vi "Swerve Wheel.vi"(8 "Wheel Angle Offset":dbl, 9 "Inputs":dbl[](array[numeric]), 10 "Pot Ref In":T1, 11 "Wheel":T3(ring)) -> (0 "Pot Ref Out":T1, 1 "Motor Output":dbl, 2 "Wheel Angle":dbl, 3 "Speed":dbl)   [LabVIEW 2018]
uses:
  <vilib>/Rock Robotics/WPI/Potentiometer/WPI_PotentiometerDevRef.ctl
  <vilib>/Rock Robotics/SystemInterfaces/AI/FPGA_AIChannel.ctl
  Drive Train Global.vi
  <vilib>/addons/control/pid/pid.llb/PID (DBL).vi
  <vilib>/addons/control/pid/NI_PID_pid.lvlib
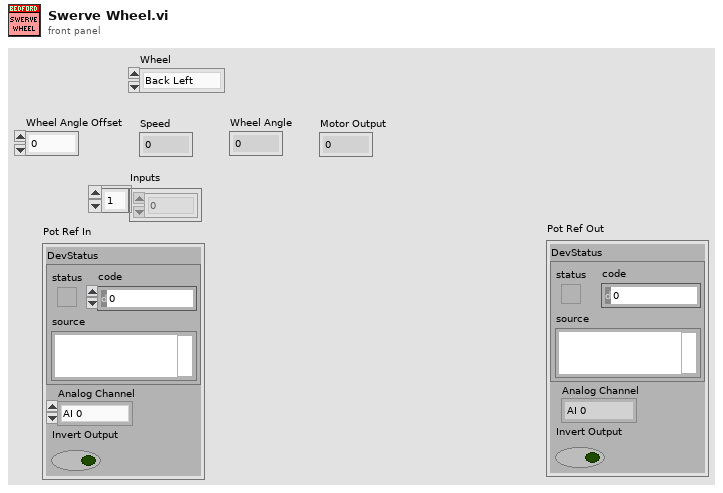
[diagram p1: front panel]
types:
  T1 = typedef "WPI_PotentiometerDevRef.ctl" = cluster{"DevStatus":errorcluster, "Analog Channel":T2, "Invert Output":bool}
  T2 = typedef "FPGA_AIChannel.ctl" = enum8{"AI 0", "AI 1", "AI 2", "AI 3", "AI MXP 0", "AI MXP 1", "AI MXP 2", "AI MXP 3", "Invalid"}
  T3 = enum16{"Back Left", "Back Right", "Front Left", "Front Right"}
  T4 = cluster{"proportional gain (Kc)":dbl, "integral time (Ti, min)":dbl, "derivative time (Td, min)":dbl}
  T5 = enum16{"Z", "Y", "X", "Rot. Point X", "Rot. Point Y", "Width/2", "Max", "Length/2"}
  T6 = enum16{"Z Axis", "Y", "X", "Rot. Point X", "Rot. Point Y", "Width/2", "Max", "Length/2"}
  T7 = cluster{"Front Left":cluster{"P Value":dbl, "I Value":dbl, "D Value":dbl}, "Front Right":cluster{"P Value":dbl, "I Value":dbl, "D Value":dbl}, "Back Left":cluster{"P Value":dbl, "I Value":dbl, "D Value":dbl}, "Back Right":cluster{"P Value":dbl, "I Value":dbl, "D Value":dbl}}
  T8 = cluster{"P Value":dbl, "I Value":dbl, "D Value":dbl}
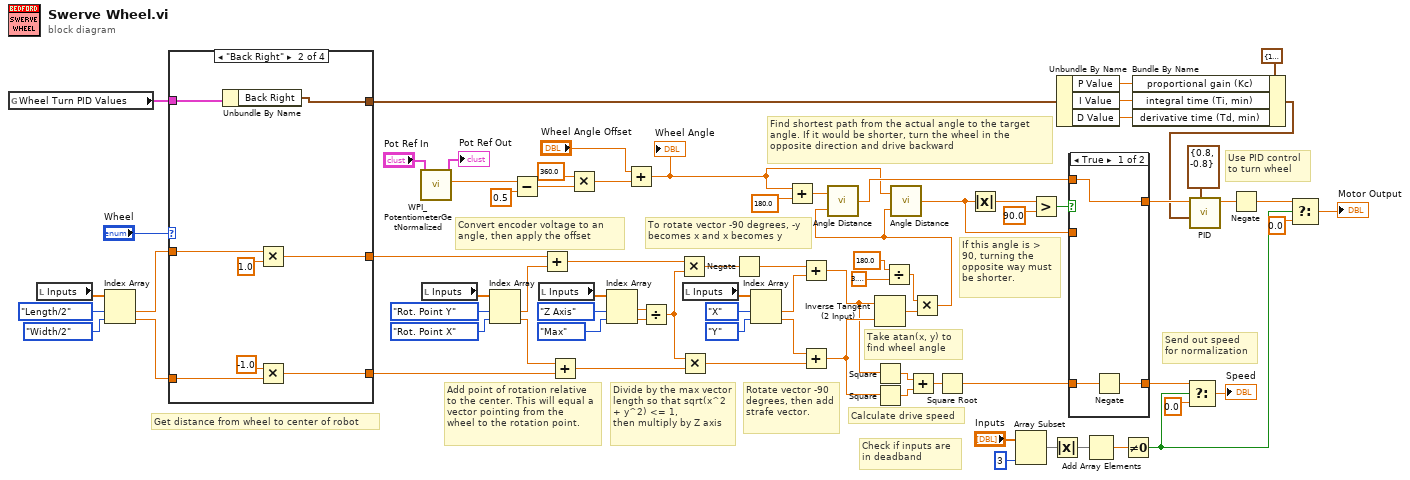
[diagram p0: block diagram]
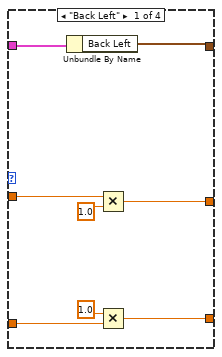
[diagram p3: hidden frame]
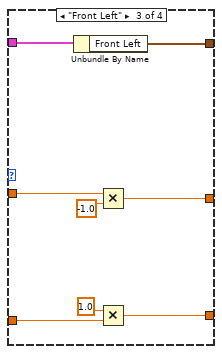
[diagram p4: hidden frame]
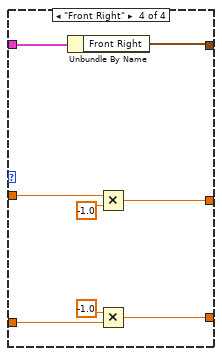
[diagram p5: hidden frame]
diagram:
  # "To rotate vector -90 degrees, -y becomes x and x becomes y"
  # "Divide by the max vector length so that sqrt(x^2 + y^2) <= 1,\nthen multiply by Z axis"
  # "Add point of rotation relative to the center. This will equal a vector pointing from the\nwheel to the rotation point."
  # "Send out speed\nfor normalization"
  # "Check if inputs are\nin deadband"
  # "Convert encoder voltage to an angle, then apply the offset"
  # "If this angle is > 90, turning the opposite way must be shorter."
  # "Use PID control\nto turn wheel"
  # "Find shortest path from the actual angle to the target angle. If it would be shorter, turn the wheel in the opposite direction and drive backward"
  # "Take atan(x, y) to find wheel angle"
  # "Calculate drive speed"
  # "Rotate vector -90 degrees, then add strafe vector."
  # "Get distance from wheel to center of robot"
  n1 = global read "Drive Train Global.vi" "Wheel Turn PID Values"() -> (w8:T7)
  n2 = local read "Inputs"() -> (w24:dbl[])
  n3 = Index Array(array=w24, index #1=T5."Length/2", index #2=T5."Width/2") -> (element #1=w22:dbl, element #2=w21:dbl)
  n4 = case shown="\"Back Right\"" "Wheel" {
    tunnel: w22 -> [w85 w93 w101 w109]
    tunnel: w21 -> [w83 w91 w99 w107]
    tunnel: [w82 w90 w98 w106] -> w48
    tunnel: [w81 w89 w97 w105] -> w44
    tunnel: w8 -> [w80 w88 w96 w104]
    tunnel: [w79 w87 w95 w103] -> w7
    frame "Back Left" {
      n5 = Unbundle By Name(w80) -> ("Back Left"=w79:T8)
      n6 = Multiply(x=w85, y=1.0) -> (x*y=w82:dbl)
      n7 = Multiply(x=1.0 ("y"), y=w83) -> (x*y=w81:dbl)
    }
    frame "Back Right" {
      n8 = Unbundle By Name(w88) -> ("Back Right"=w87:T8)
      n9 = Multiply(x=w93, y=1.0) -> (x*y=w90:dbl)
      n10 = Multiply(x=-1.0 ("y"), y=w91) -> (x*y=w89:dbl)
    }
    frame "Front Left" {
      n11 = Unbundle By Name(w96) -> ("Front Left"=w95:T8)
      n12 = Multiply(x=w101, y=-1.0) -> (x*y=w98:dbl)
      n13 = Multiply(x=1.0 ("y"), y=w99) -> (x*y=w97:dbl)
    }
    frame "Front Right" {
      n14 = Unbundle By Name(w104) -> ("Front Right"=w103:T8)
      n15 = Multiply(x=w109, y=-1.0) -> (x*y=w106:dbl)
      n16 = Multiply(x=-1.0 ("y"), y=w107) -> (x*y=w105:dbl)
    }
  }
  n17 = call <vilib>:"WPI_PotentiometerGetNormalized.vi"("PotDevRef"="Pot Ref In") -> ("Normalized Value"=w62:dbl, "PotDevRef"=→"Pot Ref Out":T1)  [unwired: 8 in, 1 out]
  n18 = local read "Inputs"() -> (w46:dbl[])
  n19 = Index Array(array=w46, index #1=T5."Rot. Point Y", index #2=T5."Rot. Point X") -> (element #1=w42:dbl, element #2=w43:dbl)
  n20 = Subtract(x=w62, y=0.5) -> (x-y=w61:dbl)
  n21 = local read "Inputs"() -> (w40:dbl[])
  n22 = Add(x=w48, y=w42) -> (x+y=w17:dbl)
  n23 = Add(x=w43, y=w44) -> (x+y=w36:dbl)
  n24 = Multiply(x=360.0 ("y"), y=w61) -> (x*y=w11:dbl)
  n25 = Index Array(array=w40, index #1=T6."Z Axis", index #2=T5."Max") -> (element #1=w37:dbl, element #2=w38:dbl)
  n26 = Add(x="Wheel Angle Offset", y=w11) -> (x+y=w13:dbl)
  "Wheel Angle" <- w13
  n27 = Divide(x=w37, y=w38) -> (x/y=w35:dbl)
  n28 = Multiply(x=w17, y=w35) -> (x*y=w19:dbl)
  n29 = Multiply(x=w35, y=w36) -> (x*y=w30:dbl)
  n30 = local read "Inputs"() -> (w33:dbl[])
  n31 = Negate(x=w19) -> (-x=w18:dbl)
  n32 = Index Array(array=w33, index #1=T5."X", index #2=T5."Y") -> (element #1=w28:dbl, element #2=w29:dbl)
  n33 = Add(x=w13, y=180.0 ("f")) -> (x+y=w57:dbl)
  n34 = Add(x=w18, y=w28) -> (x+y=w26:dbl)
  n35 = Add(x=w29, y=w30) -> (x+y=w27:dbl)
  n36 = Inverse Tangent (2 Input)(1:w27, 2:w26) -> (0:w75:dbl)
  n37 = Square(x=w26) -> (x^2=w31:dbl)
  n38 = Square(x=w27) -> (x^2=w74:dbl)
  n39 = Divide(x=180.0 ("y"), y=3.141592653589793) -> (x/y=w72:dbl)
  n40 = Add(x=w31, y=w74) -> (x+y=w73:dbl)
  n41 = Multiply(x=w72, y=w75) -> (x*y=w20:dbl)
  n42 = call "Angle Distance.vi"("target angle"=w20, "current angle"=w57) -> ("distance"=w15:dbl)
  n43 = call "Angle Distance.vi"("target angle"=w20, "current angle"=w13) -> ("distance"=w67:dbl)
  n44 = Square Root(x=w73) -> (sqrt(x)=w66:dbl)
  n45 = Absolute Value(x=w67) -> (abs(x)=w68:dbl)
  n46 = Array Subset(array="Inputs", length=3) -> (w56:dbl[])  [unwired: 1 in]
  n47 = Greater?(x=w68, y=90.0) -> (0:w52:bool)
  n48 = Absolute Value(x=w56) -> (abs(x)=w49:dbl[])
  n49 = Unbundle By Name(w7) -> ("P Value"=w6:dbl, "I Value"=w4:dbl, "D Value"=w3:dbl)
  n50 = case shown="True" w52 {
    tunnel: w15 -> [w111 _]
    tunnel: w67 -> [_ w115]
    tunnel: [w112 w114] -> w55
    tunnel: w66 -> [w113 w114]
    tunnel: [w111 w115] -> w64
    frame True {
      n51 = Negate(x=w113) -> (-x=w112:dbl)
    }
    frame False {
    }
  }
  n52 = Add Array Elements(numeric array=w49) -> (sum=w76:dbl)
  n53 = Not Equal To 0?(x=w76) -> (x != 0?=w51:bool)
  n54 = Bundle By Name(cluster=T4 {"proportional gain (Kc)"=1.0, "integral time (Ti, min)"=0.01, "derivative time (Td, min)"=0.0} ("PID gains"), "proportional gain (Kc)"=w6, "integral time (Ti, min)"=w4, "derivative time (Td, min)"=w3) -> (w2:T4)
  n55 = Select(t=w55, s=w51, f=0.0) -> (s? t:f=→"Speed":dbl)
  n56 = call-poly <vilib>:"PID.vi"("output range"=cluster{"output high":dbl, "output low":dbl} {"output high"=0.8, "output low"=-0.8}, "PID gains"=w2, "setpoint"=w64) -> ("output"=w59:dbl)  [unwired: 7 in, 1 out]
  n57 = Negate(x=w59) -> (-x=w50:dbl)
  n58 = Select(t=w50, s=w51, f=0.0) -> (s? t:f=→"Motor Output":dbl)
